vi "Neocera21 Set T -V1.vi"(5 "Channel":i16=1, 6 "Ramp rate, K/min":dbl=0.03, 8 "error in (no error)":errorcluster, 9 "Approach":T1, 10 "Set T":dbl=21.0, 11 "VISA Resource Name":refnum<visa-resource-name>="GPIB0::15::INSTR") -> (0 "error out":errorcluster, 3 "VISA Resource Name Out":refnum<visa-resource-name>)   [LabVIEW 2015]
uses:
  Instruments/Neocera/Neocera Set Point Aproach.ctl
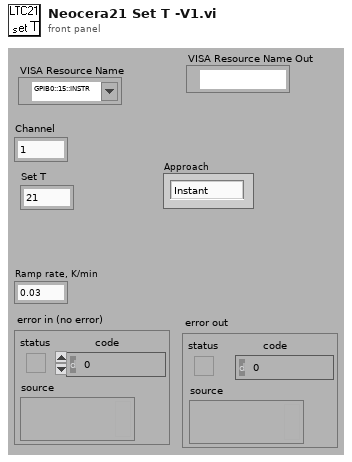
[diagram p1: front panel]
types:
  T1 = typedef "Neocera Set Point Aproach.ctl" = enum16{"Instant", "Ramp"}
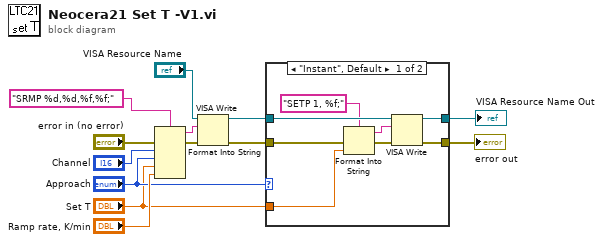
[diagram p0: block diagram]
diagram:
  n1 = Format Into String(format string="SRMP %d,%d,%f,%f;" ("data string"), error in="error in (no error)", "Channel", "Approach", "Set T", "Ramp rate, K/min") -> (resulting string=w10:string, error out=w11:errorcluster)  [unwired: 1 in]
  n2 = VISA Write(VISA resource name="VISA Resource Name", write buffer=w10, error in (no error)=w11) -> (VISA resource name out=w3:refnum<visa-resource-name>, error out=w5:errorcluster)  [unwired: 1 out]
  n3 = case shown="\"Instant\", Default" "Approach" {
    tunnel: w5 -> [w21 w23]
    tunnel: [w20 w23] -> w4
    tunnel: w3 -> [w19 w22]
    tunnel: [w18 w22] -> w2
    tunnel: "Set T" -> [w14 _]
    frame "Instant", Default {
      n4 = Format Into String(format string="SETP 1, %f;", error in=w21, w14) -> (resulting string=w15:string, error out=w17:errorcluster)  [unwired: 1 in]
      n5 = VISA Write(VISA resource name=w19, write buffer=w15, error in (no error)=w17) -> (VISA resource name out=w18:refnum<visa-resource-name>, error out=w20:errorcluster)  [unwired: 1 out]
    }
    frame "Ramp" {
    }
  }
  "error out" <- w4
  "VISA Resource Name Out" <- w2
